vi "VGap_Gap Change.vi"() -> ()   [LabVIEW 2010]
panel:
  out "error out":errorcluster
  in  "Step Change (um)":i32
  in  "Gap Change (um)":i32
  in  "error in (no error)":errorcluster
  in  "MCS System Locator":string
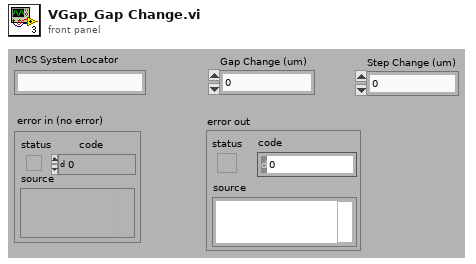
[diagram p1: front panel]
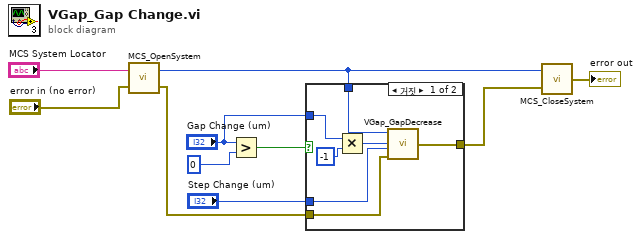
[diagram p0: block diagram]
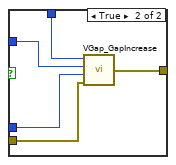
[diagram p2: hidden frame]
diagram:
  n1 = call "MCS_OpenSystem.vi"("error in (no error)"="error in (no error)", "MCS System Locator"="MCS System Locator") -> ("error out"=w2:errorcluster, "System Index Out"=w4:u32)
  n2 = Greater?(x="Gap Change (um)", y=0) -> (0:w6:bool)
  n3 = case shown="거짓" w6 {
    tunnel: "Gap Change (um)" -> [w13 w21]
    tunnel: w4 -> [w16 w22]
    tunnel: "Step Change (um)" -> [w14 w20]
    tunnel: w2 -> [w15 w19]
    tunnel: [w17 w18] -> w1
    frame False {
      n4 = Multiply(x=w13, y=-1) -> (x*y=w12:i32)
      n5 = call "VGap_GapDecrease.vi"("error in (no error)"=w15, "Step Decrease (um)"=w14, "Gap Decrease (um)"=w12, "System Index In"=w16) -> ("error out"=w17:errorcluster)
    }
    frame True {
      n6 = call "VGap_GapIncrease.vi"("error in (no error)"=w19, "Step Increase (um)"=w20, "Gap Increase (um)"=w21, "System Index In"=w22) -> ("error out"=w18:errorcluster)
    }
  }
  n7 = call "MCS_CloseSystem.vi"("error in (no error)"=w1, "System Index In"=w4) -> ("error out"=→"error out":errorcluster)
